vi "Get Gesture Data.vi"(11 "gesture in":refnum<class "Gesture.lvclass">) -> (0 "offset":T1, 1 "point":T1, 2 "gesture":T2, 3 "gesture out":refnum<class "Gesture.lvclass">, 4 "elapsed time":u32)   [LabVIEW 2023, in "Gesture.lvclass"]
doc: "Retrieve the private data from the Gesture object."
uses:
  Gesture.lvclass
  Gesture Enum.ctl
  <vilib>/Utility/miscctls.llb/LVPoint32TypeDef.ctl
  Gesture.lvclass/Gesture.ctl
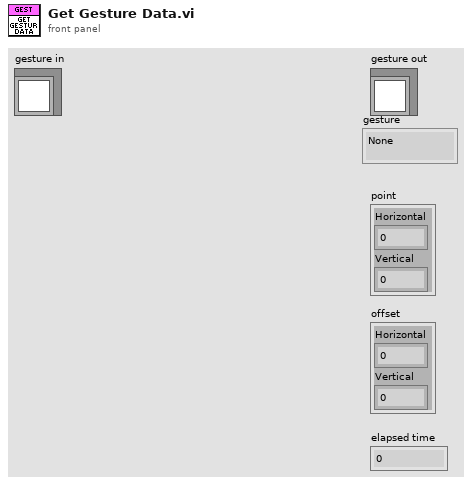
[diagram p1: front panel]
types:
  T1 = typedef "LVPoint32TypeDef.ctl" = cluster{"Horizontal":i32, "Vertical":i32}
  T2 = typedef "Gesture.lvclass/Gesture Enum.ctl" = enum16{"None", "Stop", "Tap", "Press", "Pan Start", "Pan Continue", "Pan End", "Pinch Open", "Pinch Close", "Double Tap"}
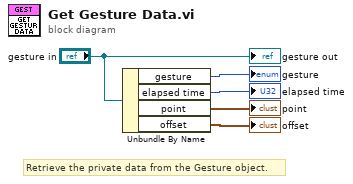
[diagram p0: block diagram]
diagram:
  # "Retrieve the private data from the Gesture object."
  n1 = Unbundle By Name("gesture in") -> ("gesture"=→"gesture":T2, "elapsed time"=→"elapsed time":u32, "point"=→"point":T1, "offset"=→"offset":T1)
  "gesture out" <- "gesture in"
